vi "Get All Library Classes.vi"(8 "error in (no error)":errorcluster, 11 "library ref":refnum<vi>) -> (0 "error out":errorcluster, 3 "class refs":refnum<vi>[](array[refnum]))   [LabVIEW 2017, in "Build Automation.lvlib"]
uses:
  Build Automation.lvlib
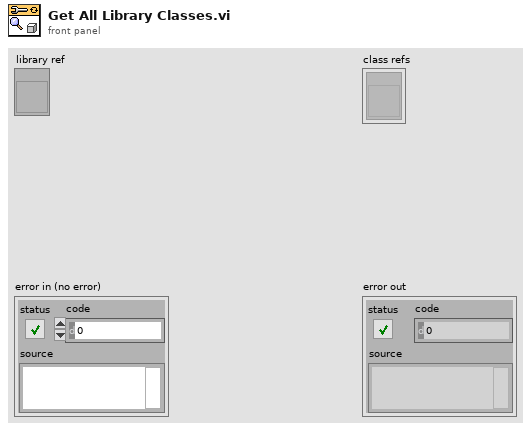
[diagram p1: front panel]
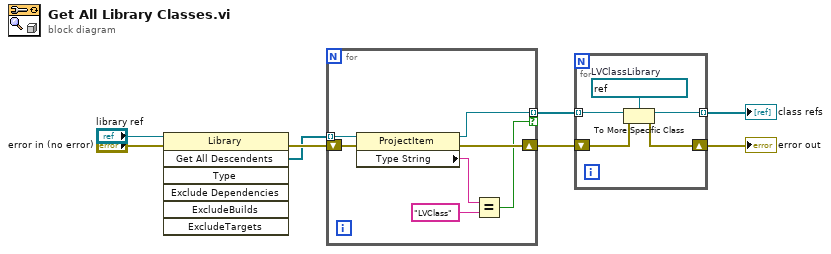
[diagram p0: block diagram]
diagram:
  n1 = invoke class="Library" method="Get All Descendents"(reference="library ref", error in="error in (no error)") -> (error out=w7:errorcluster, "All Descendents"=w6:refnum<vi>[])  [unwired: 5 in, 5 out]
  n2 = for {
    tunnel: w6 -> [w15] mode=indexing
    shift-right: [w12] -> w4
    shift-left: w7 -> [w13]
    tunnel: [w9] -> w2 mode=indexing if=w10
    n3 = property class="ProjectItem"(reference=w15, error in=w13) -> (reference out=w9:refnum<vi>, error out=w12:errorcluster, "Type String"=w11:string)
    n4 = Equal?(x=w11, y="LVClass") -> (x = y?=w10:bool)
  }
  n5 = for {
    shift-right: [w17] -> w3
    shift-left: w4 -> [w18]
    tunnel: w2 -> [w20] mode=indexing
    tunnel: [w16] -> w1 mode=indexing
    w19 = refnum<vi> refnum  # LVClassLibrary
    n6 = To More Specific Class(target class=w19, reference=w20, error in=w18) -> (specific class reference=w16:refnum<vi>, error out=w17:errorcluster)
  }
  "error out" <- w3
  "class refs" <- w1
